vi "Client Demo.vi"() -> ()   [LabVIEW 2024]
uses:
  NATS Client/NATS Client.lvclass
  NATS Subscription/NATS Subscription.lvclass
  Controls/msg type.ctl
  NATS Core.lvlib
  Controls/nats message.ctl
panel:
  in  "Tab Control":enum32{"sub", "unsub", "request"}(tab)
  in  "sub":bool
  in  "subject":string
  out "Subscription Responses":T3(array[cluster])
  in  "subscribed subjects":u16(ring) items=["", "test.whammy", "test.whammy", "test.whammy"]
  in  "unsub":bool
  in  "request":bool
  out "response":T1
  in  "request subject":string
  in  "reply subject":string="wham.whoop"
  in  "payload":string
  out "error out":errorcluster
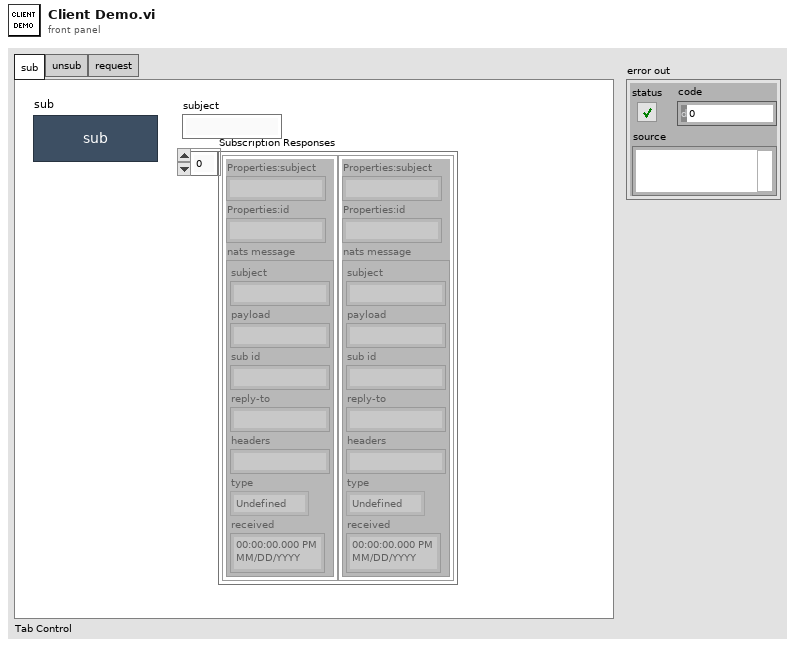
[diagram p1: front panel]
types:
  T1 = typedef "NATS Core.lvlib/nats message.ctl" = cluster{"subject":string, "payload":string, "sub id":string, "reply-to":string, "headers":string, "type":T2, "received":timestamp}
  T2 = typedef "NATS Core.lvlib/msg type.ctl" = enum16{"Undefined", "MSG", "HMSG", "+OK", "PING", "PONG", "-ERR", "INFO"}
  T3 = cluster{"Properties:subject":string, "Properties:id":string, "nats message":T1}[]
  T4 = cluster{"Properties:subject":string, "Properties:id":string, "nats message":T1}
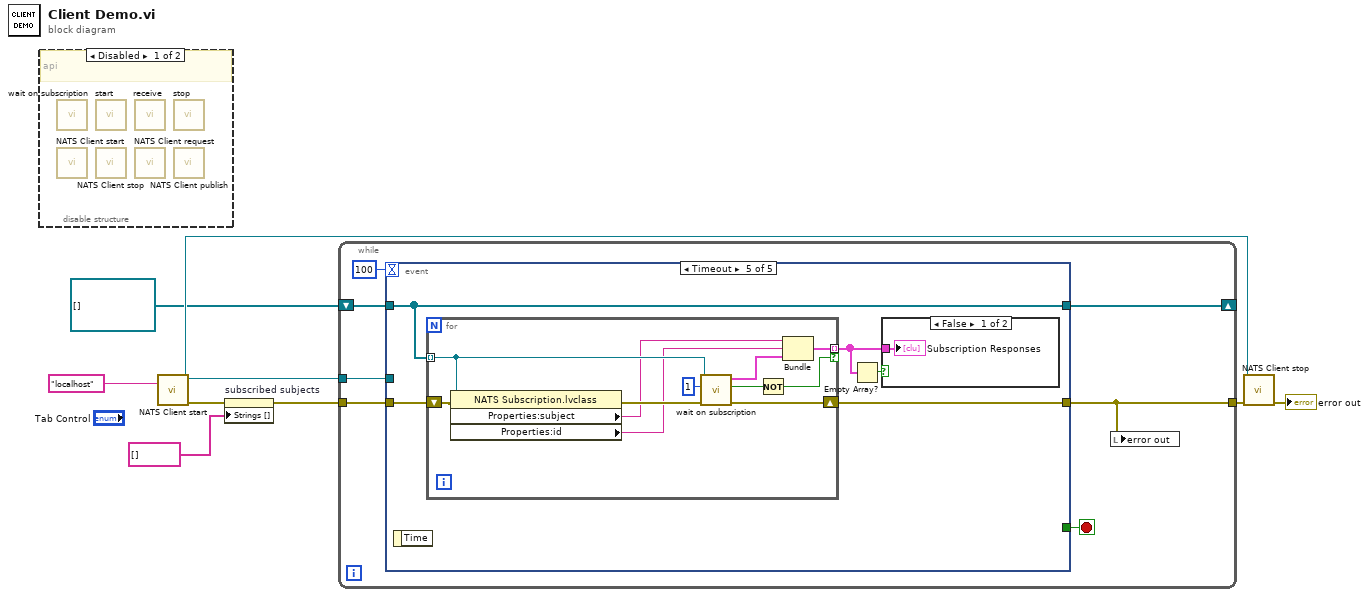
[diagram p0: block diagram]
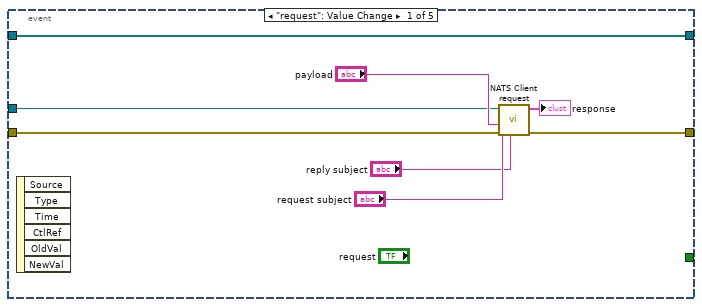
[diagram p3: hidden frame]
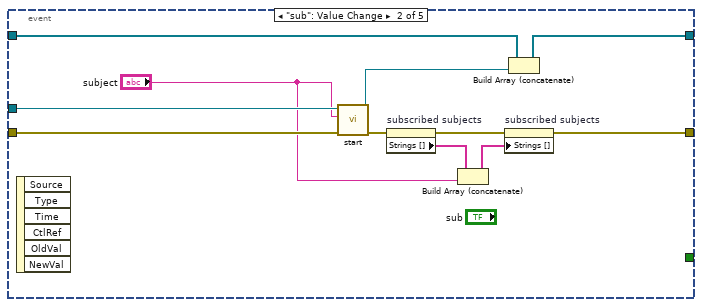
[diagram p4: hidden frame]
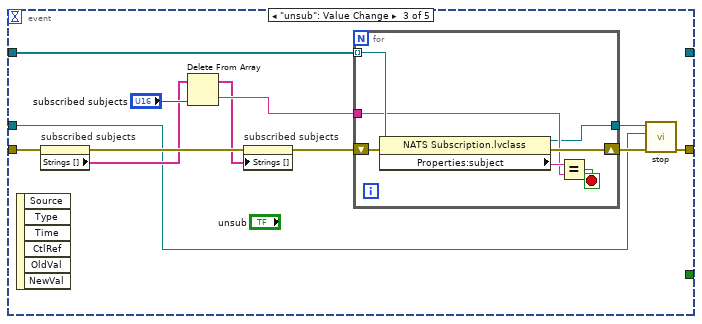
[diagram p5: hidden frame]
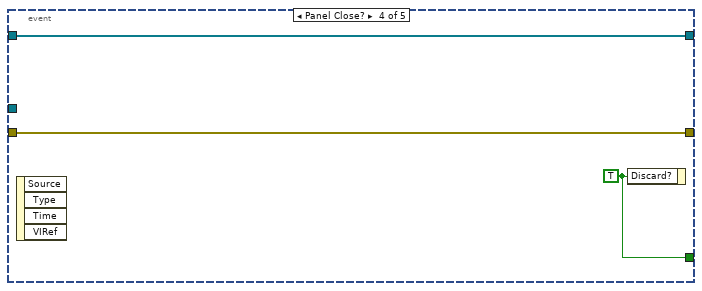
[diagram p6: hidden frame]
diagram:
  n1 = disable-structure shown="Disabled" {
    frame Disabled {
      # "api"
      n2 = call-dynamic "wait on subscription.vi"() -> ()  [unwired: 9 in, 3 out]
      n3 = call "NATS Client start.vi"() -> ()  [unwired: 10 in, 2 out]
      n4 = call "start.vi"() -> ()  [unwired: 10 in, 2 out]
      n5 = call "NATS Client stop.vi"() -> ()  [unwired: 11 in, 1 out]
      n6 = call-dynamic "receive.vi"() -> ()  [unwired: 10 in, 2 out]
      n7 = call "NATS Client request.vi"() -> ()  [unwired: 9 in, 3 out]
      n8 = call "stop.vi"() -> ()  [unwired: 11 in, 1 out]
      n9 = call "NATS Client publish.vi"() -> ()  [unwired: 11 in, 1 out]
    }
    frame Enabled {
    }
  }
  n10 = call "NATS Client start.vi"("address"="localhost") -> ("error out"=w8:errorcluster, "NATS Client out"=w3:refnum<class "NATS Client.lvclass">)  [unwired: 9 in]
  n11 = property on="subscribed subjects" class="Ring (strict)"(error in=w8, "Strings []"=string[] []) -> (error out=w5:errorcluster)  [unwired: 1 in, 1 out]
  n12 = while {
    tunnel: w5 -> [w15]
    tunnel: [w14] -> w6
    tunnel: w3 -> [w12]
    shift-right: [w10] -> _
    shift-left: refnum<class "NATS Subscription.lvclass">[] [] ("NATS Subscription") -> [w9]
    stop <- w13 stop-if-true
    n13 = event shown="[4] Timeout" {
      selector: _ -> [_ _ _ _ _]
      dyn-events: _ -> [_ _ _ _ _]
      timeout: 100 -> [_ _ _ _ _]
      tunnel: [_ _ _ w55 _] -> w13
      tunnel: [w22 w31 w46 w56 w61] -> w14
      tunnel: w15 -> [w23 w34 w45 w56 w60]
      tunnel: w12 -> [w18 w30 w36 _ _]
      tunnel: [w16 w28 _ w54 w59] -> w10
      tunnel: w9 -> [w16 w29 w38 w54 w59]
      event "request": Value Change {
        n14 = event-data() -> ()  [unwired: 1 in, 6 out]
        n15 = call "NATS Client request.vi"("reply subject"="reply subject", "error in"=w23, "payload"="payload", "subject"="request subject", "NATS Client in"=w18) -> ("error out"=w22:errorcluster, "nats message"=→"response":T1)  [unwired: 4 in, 1 out]
      }
      event "sub": Value Change {
        n16 = event-data() -> ()  [unwired: 1 in, 6 out]
        n17 = call "start.vi"("error in"=w34, "subject"="subject", "NATS Client"=w30) -> ("error out"=w33:errorcluster, "NATS Subscription"=w27:refnum<class "NATS Subscription.lvclass">)  [unwired: 7 in]
        n18 = property on="subscribed subjects" class="Ring (strict)"(error in=w33) -> (error out=w32:errorcluster, "Strings []"=w26:string[])  [unwired: 1 in, 1 out]
        n19 = Build Array (concatenate)(w26, "subject") -> (w24:string[])
        n20 = property on="subscribed subjects" class="Ring (strict)"(error in=w32, "Strings []"=w24) -> (error out=w31:errorcluster)  [unwired: 1 in, 1 out]
        n21 = Build Array (concatenate)(w29, w27) -> (w28:refnum<class "NATS Subscription.lvclass">[])
      }
      event "unsub": Value Change {
        n22 = event-data() -> ()  [unwired: 1 in, 6 out]
        n23 = property on="subscribed subjects" class="Ring (strict)"(error in=w45) -> (error out=w43:errorcluster, "Strings []"=w40:string[])  [unwired: 1 in, 1 out]
        n24 = Delete From Array(array=w40, index="subscribed subjects") -> (deleted portion=w39:string, array with subset deleted=w35:string[])  [unwired: 1 in]
        n25 = property on="subscribed subjects" class="Ring (strict)"(error in=w43, "Strings []"=w35) -> (error out=w42:errorcluster)  [unwired: 1 in, 1 out]
        n26 = for {
          tunnel: w39 -> [w48]
          tunnel: w38 -> [w51] mode=indexing
          tunnel: [w47] -> w37
          shift-right: [w52] -> w44
          shift-left: w42 -> [w53]
          stop <- w49 stop-if-true
          n27 = property class="NATS Subscription.lvclass"(reference=w51, error in=w53) -> (reference out=w47:refnum<class "NATS Subscription.lvclass">, error out=w52:errorcluster, "Properties:subject"=w50:string)
          n28 = Equal?(x=w50, y=w48) -> (x = y?=w49:bool)
        }
        n29 = call "stop.vi"("error in"=w44, "NATS Client"=w36, "NATS Subscription"=w37) -> ("error out"=w46:errorcluster)  [unwired: 8 in]
      }
      event Panel Close? {
        w55 = TRUE ("Discard?")
        n30 = event-data() -> ()  [unwired: 1 in, 4 out]
        n31 = event-data("Discard?"=w55) -> ()  [unwired: 1 in, 1 out]
      }
      event Timeout {
        n32 = event-data() -> ()  [unwired: 1 in, 1 out]
        n33 = for {
          tunnel: w59 -> [w69] mode=indexing
          shift-right: [w73] -> w61
          shift-left: w60 -> [w71]
          tunnel: [w65] -> w58 mode=indexing if=w63
          n34 = property class="NATS Subscription.lvclass"(reference=w69, error in=w71) -> (error out=w72:errorcluster, "Properties:subject"=w66:string, "Properties:id"=w67:string)  [unwired: 1 out]
          n35 = call-dynamic "wait on subscription.vi"("error in"=w72, "timeout in ms (-1)"=1, "NATS Subscriber in"=w69) -> ("error out"=w73:errorcluster, "time out"=w64:bool, "nats message"=w68:T1)  [unwired: 6 in]
          n36 = Not(x=w64) -> (.not. x?=w63:bool)
          n37 = Bundle("Properties:subject"=w66, "Properties:id"=w67, "nats message"=w68) -> (w65:T4)  [unwired: 1 in]
        }
        n38 = Empty Array?(array=w58) -> (empty?=w57:bool)
        n39 = case shown="False" w57 {
          tunnel: w58 -> [w62 _]
          frame False {
            "Subscription Responses" <- w62
          }
          frame True {
          }
        }
      }
    }
    n40 = local write "error out"(w14) -> ()
  }
  n41 = call "NATS Client stop.vi"("error in"=w6, "NATS Client"=w3) -> ("error out"=→"error out":errorcluster)  [unwired: 9 in]
